vi "WebSlider.vi"(10 "Slider Value":dbl(slide) min=-10.0 max=10.0 step=0.1 scale=-10.0..10.0, 11 "URL":string="myweb.wit.edu/bennetts4/ELEC3800/Lab10/writeVal.php?wrVal=") -> (0 "Requests to MyWeb":i16, 1 "Slider Value to Write":dbl, 2 "Body":string, 3 "Header":string)   [LabVIEW 2017]
uses:
  <vilib>/httpClient/LabVIEWHTTPClient.lvlib
panel:
  in  "stop":bool
  out "Path":path
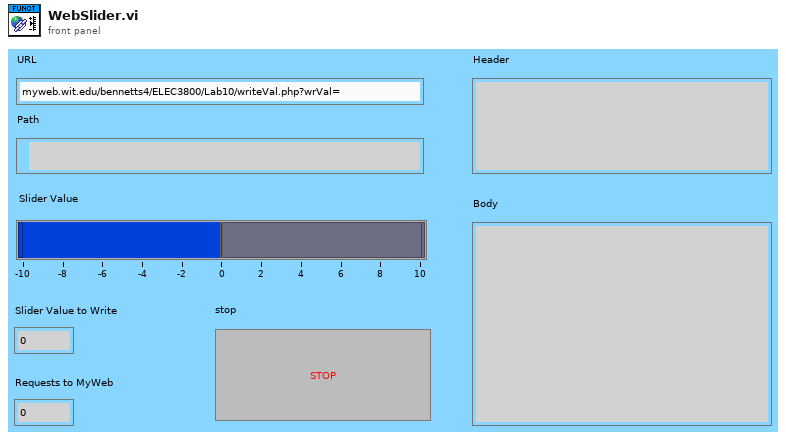
[diagram p1: front panel]
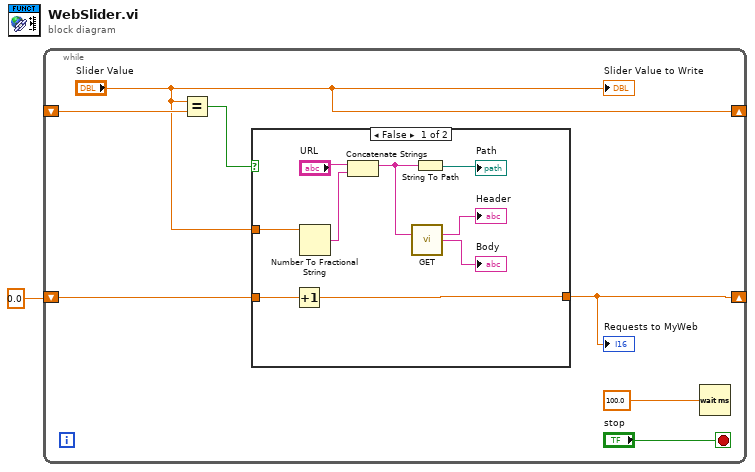
[diagram p0: block diagram]
diagram:
  n1 = while {
    shift-right: ["Slider Value"] -> _
    shift-left: _ -> [w7]
    shift-right: [w3] -> _
    shift-left: 0.0 -> [w4]
    stop <- "stop" stop-if-true
    n2 = Equal?(x="Slider Value", y=w7) -> (x = y?=w6:bool)
    n3 = case shown="False" w6 {
      tunnel: "Slider Value" -> [w11 _]
      tunnel: w4 -> [w10 w18]
      tunnel: [w9 w18] -> w3
      frame False {
        n4 = Increment(x=w10) -> (x+1=w9:dbl)
        n5 = Number To Fractional String(number=w11) -> (F-format string=w17:string)  [unwired: 3 in]
        n6 = Concatenate Strings("URL", w17) -> (w14:string)
        n7 = call <vilib>:"GET.vi"("url"=w14) -> ("headers"=→"Header":string, "body"=→"Body":string)  [unwired: 11 in, 2 out]
        n8 = String To Path(string=w14) -> (path=→"Path":path)
      }
      frame True {
      }
    }
    "Requests to MyWeb" <- w3
    n9 = Wait (ms)(milliseconds to wait=100.0) -> ()  [unwired: 1 out]
    "Slider Value to Write" <- "Slider Value"
  }
